vi "Initialize.vi"(8 "error in":errorcluster, 11 "Lv Proj Document Type:TAF Proj":refnum<class "TAF Proj.lvclass">) -> (0 "error out":errorcluster, 3 "Lv Proj Document Type:TAF Proj":refnum<class "TAF Proj.lvclass">)   [LabVIEW 2021, in "TAF Proj Document Type.lvlib" / "TAF Proj.lvclass"]
uses:
  <vilib>/Wovalab/AntiDoc/Document Type/Add-ons/LabVIEW TAF Project/TAF Proj/TAF Proj.lvclass
  C:/Program Files (x86)/National Instruments/LabVIEW 2021/vi.lib/Wovalab/AntiDoc/Document Type/Document/Document Type.lvclass
  <vilib>/Wovalab/AntiDoc/Document Type/Add-ons/LabVIEW TAF Project/TAF Proj Config/TAF Proj Config.lvclass
  <vilib>/Wovalab/AntiDoc/Document Type/Document/Document Type.lvclass/Document Type.ctl
  <vilib>/Wovalab/AntiDoc/Document Type/Add-ons/LabVIEW TAF Project/TAF Proj Config/TAF Proj Config.lvclass/TAF Proj Config.ctl
  <vilib>/Wovalab/AntiDoc/Document Type/Add-ons/LabVIEW TAF Project/TAF Proj/TAF Proj.lvclass/TAF Proj.ctl
  <vilib>/Wovalab/AntiDoc/Document Type/Document/Read Config.vi
  <vilib>/Wovalab/AntiDoc/Document Type/Add-ons/LabVIEW TAF Project/TAF Proj Config/Read Project Path.vi
  <vilib>/Wovalab/AntiDoc/Document Type/Config/Config.lvclass
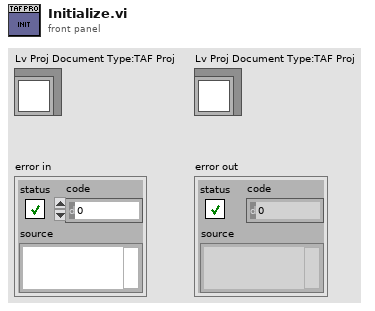
[diagram p1: front panel]
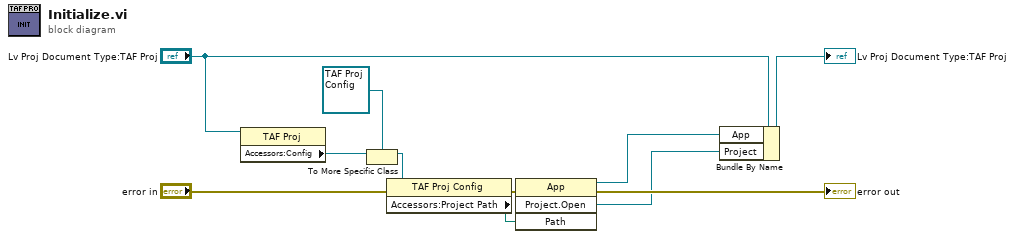
[diagram p0: block diagram]
diagram:
  n1 = property class="TAF Proj"(reference="Lv Proj Document Type:TAF Proj") -> ("Accessors:Config"=w4:refnum<class "Config.lvclass">)  [unwired: 1 in, 2 out]
  n2 = To More Specific Class(target class=refnum<class "TAF Proj Config.lvclass"> refnum ("Lv Proj Document Type.lvlib:Config"), reference=w4) -> (specific class reference=w1:refnum<class "TAF Proj Config.lvclass">)  [unwired: 1 in, 1 out]
  n3 = property class="TAF Proj Config"(reference=w1, error in="error in") -> (error out=w9:errorcluster, "Accessors:Project Path"=w6:path)  [unwired: 1 out]
  n4 = invoke class="App" method="Project.Open"(error in=w9, "Path"=w6) -> (reference out=w5:refnum<vi>, error out=→"error out":errorcluster, "Project:Open"=w7:refnum<vi>)  [unwired: 2 in, 1 out]
  n5 = Bundle By Name(cluster="Lv Proj Document Type:TAF Proj", "App"=w5, "Project"=w7) -> (→"Lv Proj Document Type:TAF Proj":refnum<class "TAF Proj.lvclass">)
